vi "Change Active Enable Symbol.vi"(8 "error in (no error)":errorcluster, 11 "Selector in":refnum<class "Selector.lvclass">) -> (0 "error out":errorcluster, 2 "Name":string, 3 "Selector out":refnum<class "Selector.lvclass">)   [LabVIEW 2019, in "Selector.lvclass"]
uses:
  Selector.lvclass
  Selector.lvclass/Selector.ctl
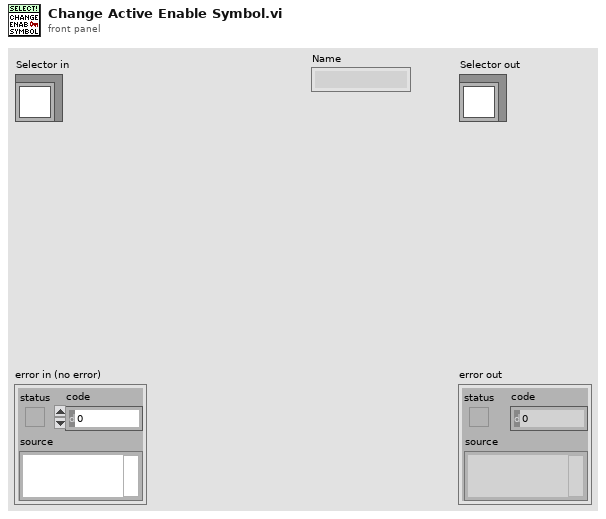
[diagram p1: front panel]
types:
  T1 = typedef "Selector.lvclass/Item.ctl" = cluster{"Name":string, "Group":string, "Enabled":bool}
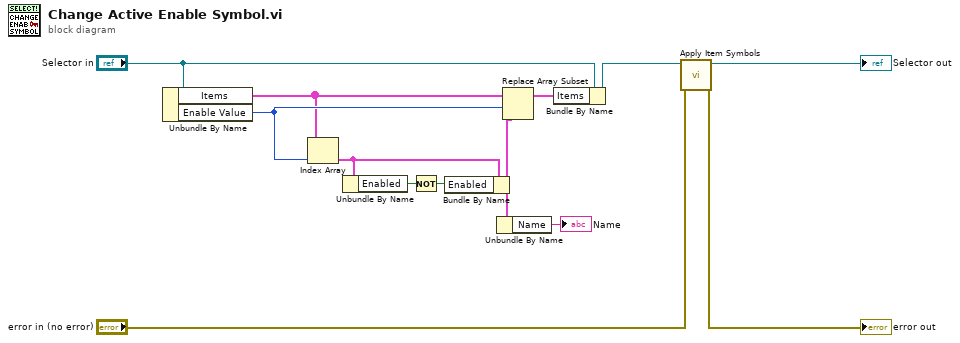
[diagram p0: block diagram]
diagram:
  n1 = Unbundle By Name("Selector in") -> ("Items"=w12:T1[], "Enable Value"=w13:i32)
  n2 = Index Array(array=w12, index=w13) -> (element=w4:T1)
  n3 = Unbundle By Name(w4) -> ("Enabled"=w5:bool)
  n4 = Not(x=w5) -> (.not. x?=w3:bool)
  n5 = Bundle By Name(cluster=w4, "Enabled"=w3) -> (w2:T1)
  n6 = Unbundle By Name(w2) -> ("Name"=→"Name":string)
  n7 = Replace Array Subset(array=w12, new element=w2, index=w13) -> (w11:T1[])
  n8 = Bundle By Name(cluster="Selector in", "Items"=w11) -> (w9:refnum<class "Selector.lvclass">)
  n9 = call-dynamic "Apply Item Symbols.vi"("error in (no error)"="error in (no error)", "Selector in"=w9) -> ("error out"=→"error out":errorcluster, "Selector out"=→"Selector out":refnum<class "Selector.lvclass">)  [unwired: 8 in]
